vi "Set Display Wash Step from User Console.vi"(8 "error in (no error)":errorcluster, 10 "Wash Steps":T1, 11 "Car Wash Controller Actor in":refnum<class "Car Wash Controller Actor.lvclass">) -> (0 "error out":errorcluster, 3 "Car Wash Controller Actor out":refnum<class "Car Wash Controller Actor.lvclass">)   [LabVIEW 2019, in "Car Wash Controller Actor.lvlib" / "Car Wash Controller Actor.lvclass"]
uses:
  Car Wash Controller Actor.lvclass
  Sim Entry Console Actor/Sim Entry Console Actor/Wash steps selection -Buttons.ctl
  Car Wash Controller Actor.lvclass/Car Wash Controller Actor.ctl
  Simulated Wash Display Console Actor/Simulated Wash Display Console Actor Messages/Update Car Wash Indicators Msg/Update Car Wash Indicators Msg.lvclass/Update Car Wash Indicators Msg.ctl
  <vilib>/ActorFramework/Message Enqueuer/Message Enqueuer.lvclass/Message Enqueuer.ctl
  <vilib>/ActorFramework/Message Enqueuer/Enqueue.vi
  Simulated Wash Display Console Actor/Simulated Wash Display Console Actor Messages/Update Car Wash Indicators Msg/Update Car Wash Indicators Msg.lvclass
  C:/Program Files (x86)/National Instruments/LabVIEW 2019/vi.lib/ActorFramework/Message/Message.lvclass
  <vilib>/ActorFramework/Message Priority Queue/Priority Enqueue.vi
  Sim Entry Console Actor/Sim Entry Console Actor/Simulated Entry Console Actor.lvclass
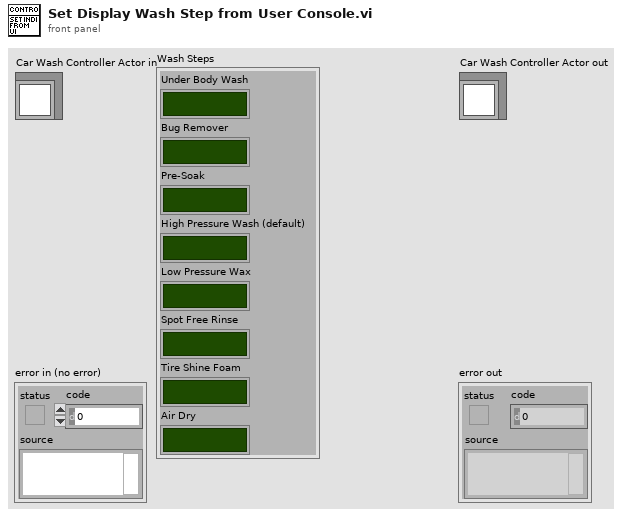
[diagram p1: front panel]
types:
  T1 = typedef "Simulated Entry Console Actor.lvlib/Simulated Entry Console Actor.lvclass/Wash steps selection -Buttons.ctl" = cluster{"Under Body Wash":bool, "Bug Remover":bool, "Pre-Soak":bool, "High Pressure Wash (default)":bool, "Low Pressure Wax":bool, "Spot Free Rinse":bool, "Tire Shine Foam":bool, "Air Dry":bool}
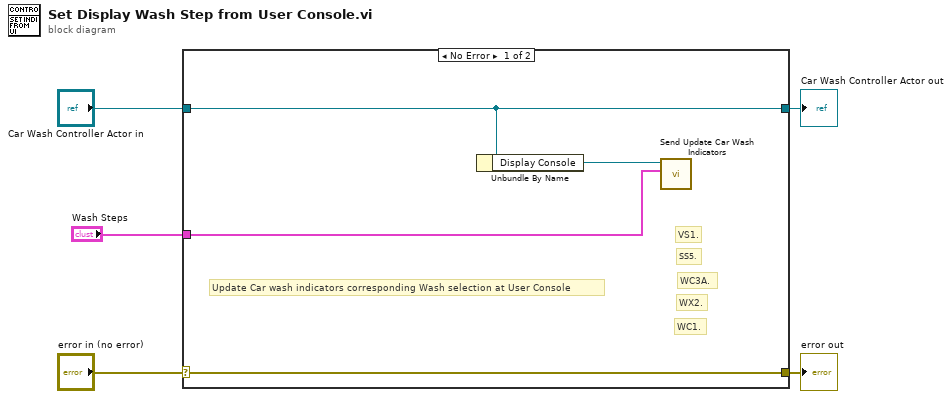
[diagram p0: block diagram]
diagram:
  n1 = case shown="No Error" "error in (no error)" {
    selector: "error in (no error)" -> [w9 w11]
    tunnel: [w9 w11] -> w4
    tunnel: [w8 w10] -> w2
    tunnel: "Car Wash Controller Actor in" -> [w8 w10]
    tunnel: "Wash Steps" -> [w6 _]
    frame No Error {
      # "WC1."
      # "WX2."
      # "WC3A."
      # "SS5."
      # "VS1."
      # "Update Car wash indicators corresponding Wash selection at User Console"
      n2 = Unbundle By Name(w8) -> ("Display Console"=w7:refnum<class "Message Enqueuer.lvclass">)
      n3 = call "Send Update Car Wash Indicators.vi"("Car Wash Indicators"=w6, "Message Enqueuer"=w7) -> ()  [unwired: 8 in, 2 out]
    }
    frame Error {
    }
  }
  "error out" <- w4
  "Car Wash Controller Actor out" <- w2
